vi "ModelCheck.vi"(8 "error in (no error)":errorcluster, 9 "ReScanNG":i32, 11 "Data In":T2) -> (0 "error out":errorcluster, 1 "States":T1, 2 "ReScanNG":i32, 3 "Data Out":T2)   [LabVIEW 2014]
uses:
  controls/Data1.ctl
  controls/Payjson.ctl
  controls/State.ctl
panel:
  out "COMPNTID":string
  out "COMPNTSN":string
  out "CheckPars":string
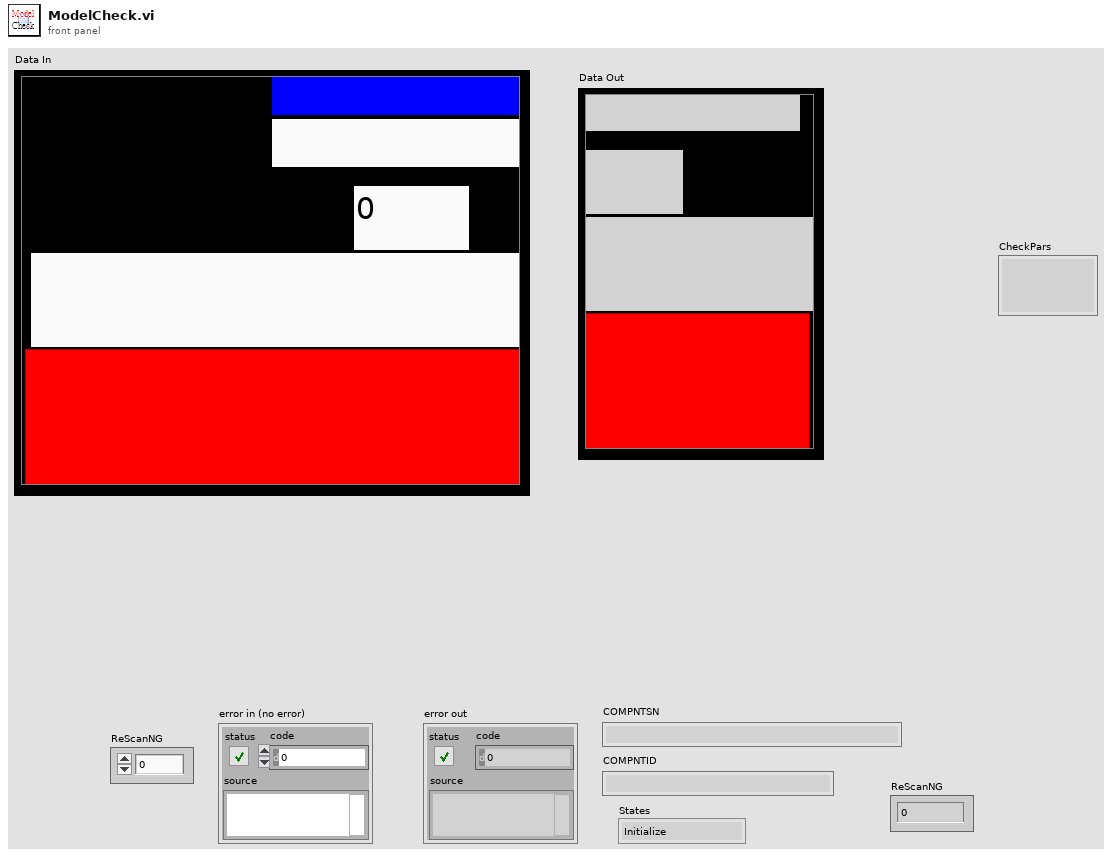
[diagram p1: front panel]
types:
  T1 = typedef "State.ctl" = enum16{"Initialize", "Wait for Scan", "State 1", "State 2", "NG", "NG1", "OK", "OKNG", "OKNG1", "Exit"}
  T2 = typedef "Data1.ctl" = cluster{"Date":string, "BarCode1":string, "BarCode2":string, "BarCode3":string, "Message":string, "OK Count":u16, "NG Count":u16, "Total Count":u16, "ModelData":string[][], "OK&NG":bool, "COM1":refnum<visa-resource-name>, "COM2":refnum<visa-resource-name>, "IO":i32, "Time":u32, "TCP":refnum<k5>, "TCP 2":refnum<k5>, "COM1 2":refnum<visa-resource-name>, "CheckNum":string, "BarCode1_1":string, "BarCode2_1":string, "BarCode3_1":string, "日期":string, "機種":string, "機號":string, "商品條碼1":string, "OK_1":string, "OK":string, "NG":string, "NG_1":string, "Total":string, "Total_1":string, "ClaerTime":u32, "Pjson":T3, "LotNo":string[], "CheckParsArray":string[], "BarCode4":string, "BarCode4_1":string, "商品條碼2":string, "BarCode5":string, "BarCode5_1":string, "商品條碼3":string}
  T3 = typedef "Payjson.ctl" = cluster{"DEPT":string, "LINE":string, "STANO":string, "WORKNO":string, "PRODSN":string, "COMPNTID":string, "COMPNTLOT":string, "COMPNTSN":string, "USEDQTY":i16, "OPDATE":string, "OPUSER":string, "RECVDATE":string, "MMODU":string}[]
  T4 = cluster{"DEPT":string, "LINE":string, "STANO":string, "WORKNO":string, "PRODSN":string, "COMPNTID":string, "COMPNTLOT":string, "COMPNTSN":string, "USEDQTY":i16, "OPDATE":string, "OPUSER":string, "RECVDATE":string, "MMODU":string}
  T5 = cluster{"DEPT":string, "LINE":string, "STANO":string, "WORKNO":string, "PRODSN":string, "COMPNTID":string, "COMPNTLOT":string, "COMPNTSN":string, "USEDQTY":i16, "OPDATE":string, "OPUSER":string, "RECVDATE":string, "MMODU":string}[]
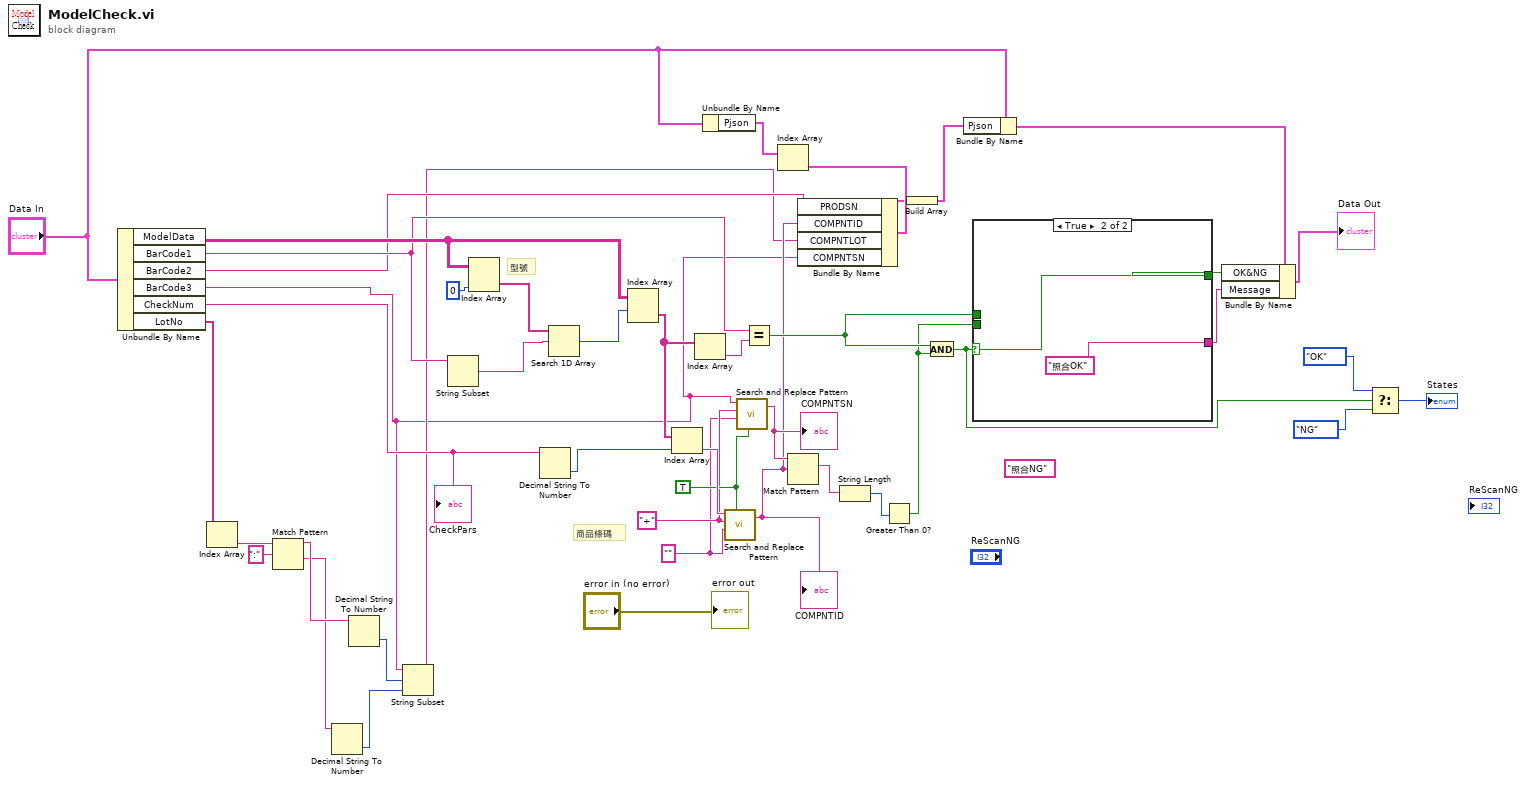
[diagram p0: block diagram]
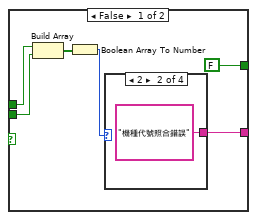
[diagram p2: hidden frame]
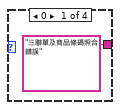
[diagram p3: hidden frame]
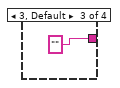
[diagram p4: hidden frame]
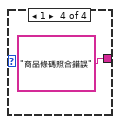
[diagram p5: hidden frame]
diagram:
  w20 = TRUE ("replace all? (F)")
  w18 = "" ("replace string (\"\")")
  w19 = "+" ("regular expression (\"\")")
  (unwired) "照合NG" ("Message")
  # "商品條碼"
  # "型號"
  n1 = Unbundle By Name("Data In") -> ("ModelData"=w42:string[][], "BarCode1"=w33:string, "BarCode2"=w11:string, "BarCode3"=w1:string, "CheckNum"=w26:string, "LotNo"=w9:string[])
  "CheckPars" <- w26
  n2 = Index Array(array=w9) -> (element=w8:string)  [unwired: 1 in]
  n3 = Match Pattern(string=w8, regular expression=":") -> (before substring=w6:string, after substring=w5:string)  [unwired: 1 in, 2 out]
  n4 = Decimal String To Number(string=w5) -> (number=w3:i32)  [unwired: 2 in, 1 out]
  n5 = Decimal String To Number(string=w6) -> (number=w4:i32)  [unwired: 2 in, 1 out]
  n6 = String Subset(string=w1, offset (0)=w4, length (rest)=w3) -> (substring=w2:string)
  n7 = String Subset(string=w33) -> (substring=w38:string)  [unwired: 2 in]
  n8 = Index Array(array=w42, index (col)=0 ("disabled index (col)")) -> (element=w43:string[])  [unwired: 1 in]
  n9 = Decimal String To Number(string=w26) -> (number=w28:i32)  [unwired: 2 in, 1 out]
  n10 = Search 1D Array(1D array=w43, element=w38) -> (index of element=w37:i32)  [unwired: 1 in]
  n11 = Index Array(array=w42, index (row)=w37) -> (element=w29:string[])  [unwired: 1 in]
  n12 = Index Array(array=w29, index=w28) -> (element=w22:string)
  n13 = Index Array(array=w29) -> (element=w36:string)  [unwired: 1 in]
  n14 = Unbundle By Name("Data In") -> ("Pjson"=w15:T3)
  n15 = call <vilib>:"Search and Replace Pattern.vi"("string"=w22, "regular expression (\"\")"=w19, "replace string (\"\")"=w18, "replace all? (F)"=w20) -> ("result string"=w10:string)  [unwired: 1 in, 1 out]
  "COMPNTID" <- w10
  n16 = call <vilib>:"Search and Replace Pattern.vi"("string"=w1, "regular expression (\"\")"=w19, "replace string (\"\")"=w18, "replace all? (F)"=w20) -> ("result string"=w21:string)  [unwired: 1 in, 1 out]
  "COMPNTSN" <- w21
  n17 = Equal?(x=w33, y=w36) -> (x = y?=w34:bool)
  n18 = Index Array(array=w15) -> (element=w14:T4)  [unwired: 1 in]
  n19 = Match Pattern(string=w21, regular expression=w10) -> (match substring=w25:string)  [unwired: 1 in, 3 out]
  n20 = Bundle By Name(cluster=w14, "PRODSN"=w11, "COMPNTID"=w10, "COMPNTLOT"=w2, "COMPNTSN"=w1) -> (w13:T4)
  n21 = String Length(string=w25) -> (length=w24:i32)
  n22 = Greater Than 0?(x=w24) -> (x > 0?=w23:bool)
  n23 = Build Array(w13) -> (w12:T5)
  n24 = And(x=w34, y=w23) -> (x .and. y?=w30:bool)
  n25 = Bundle By Name(cluster="Data In", "Pjson"=w12) -> (w17:T2)
  n26 = case shown="True" w30 {
    selector: w30 -> [_ w56]
    tunnel: [FALSE w56] -> w41
    tunnel: [w45 "照合OK" ("Message")] -> w35
    tunnel: w34 -> [w50 _]
    tunnel: w23 -> [w49 _]
    frame False {
      n27 = Build Array(w50, w49) -> (w48:bool[])
      n28 = Boolean Array To Number(Boolean array=w48) -> (number=w46:u32)
      n29 = case shown="2" w46 {
        tunnel: ["三聯單及商品條碼照合錯誤" "機種代號照合錯誤" "" "商品條碼照合錯誤"] -> w45
        frame 0 {
        }
        frame 2 {
        }
        frame 3, Default {
        }
        frame 1 {
        }
      }
    }
    frame True {
    }
  }
  n30 = Bundle By Name(cluster=w17, "OK&NG"=w41, "Message"=w35) -> (→"Data Out":T2)
  n31 = Select(t=State."OK" ("States"), s=w30, f=State."NG" ("States")) -> (s? t:f=→"States":T1)
  "error out" <- "error in (no error)"
